vi "simulation_freq_MRC.vi"() -> ()   [LabVIEW 2014] (continued)
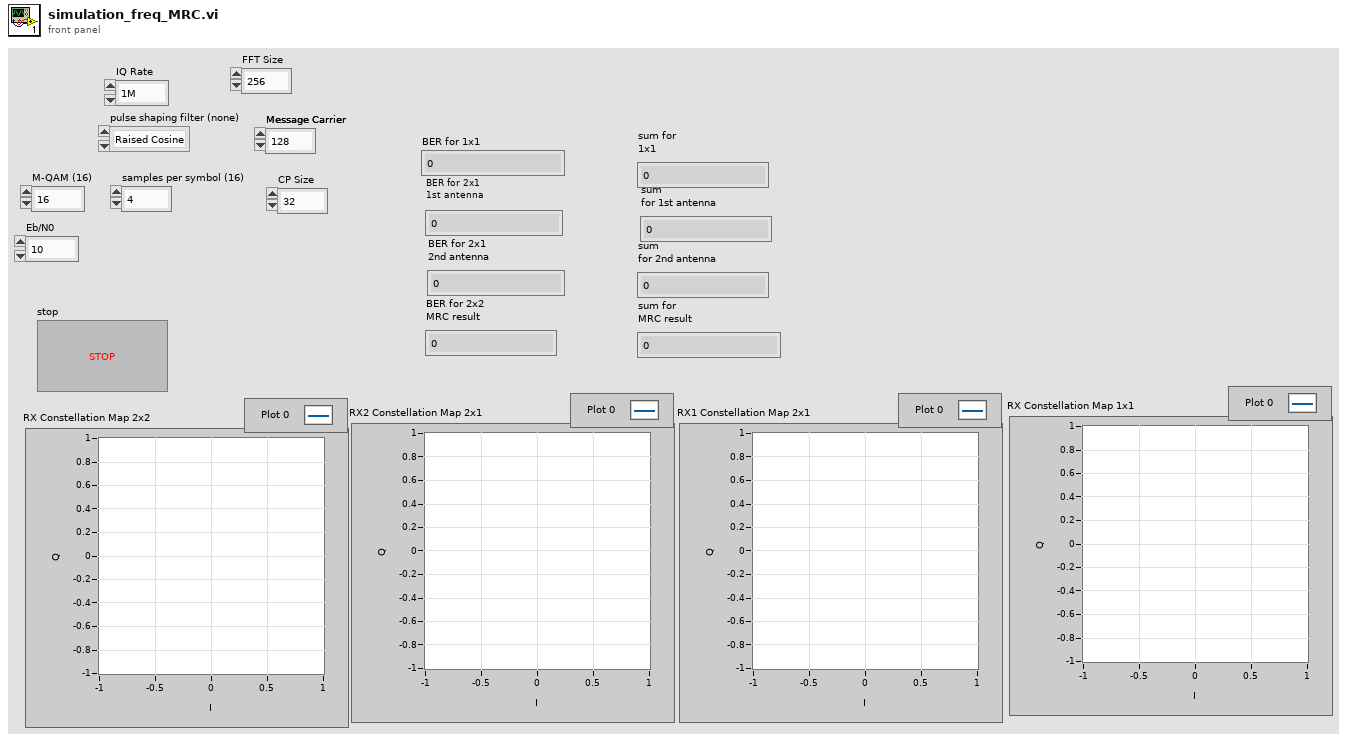
[diagram p1: front panel]
types:
  T1 = enum16{"none", "Raised Cosine", "Root Raised Cos", "Gaussian"}
  T2 = enum16{"FSK", "PSK", "QAM", "MSK", "PAM", "ASK", "CPM"}
  T3 = cluster{"samples per symbol (16)":i32, "symbol map":cdb[]}
  T4 = typedef "niAMT.lvlib/Complex Data Waveform.ctl" = cluster{"t0":dbl, "dt":dbl, "Y":cdb[]}
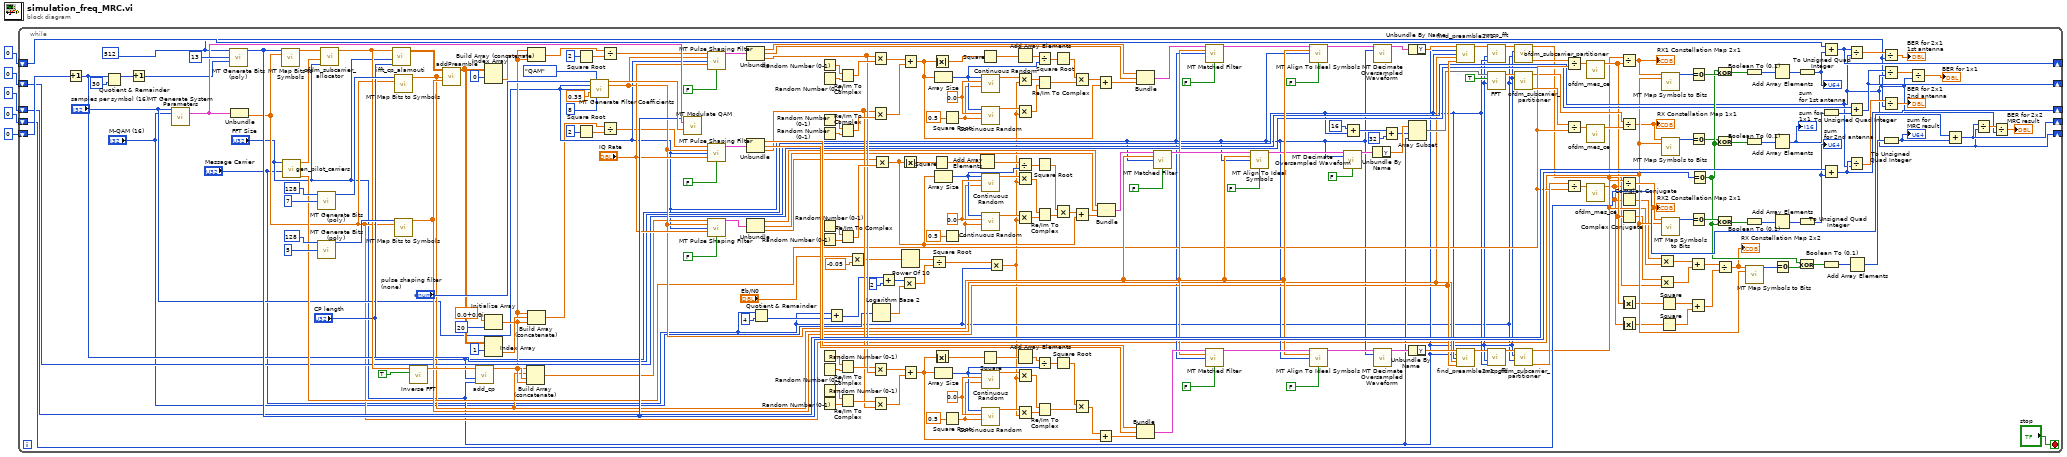
[diagram p0: block diagram]
diagram:
  n1 = while {
    shift-right: [w130] -> _
    shift-left: u64 0 -> [w214]
    shift-right: [w70] -> _
    shift-left: u64 0 -> [w215]
    shift-right: [w133] -> _
    shift-left: u64 0 -> [w178]
    shift-right: [w127] -> _
    shift-left: u64 0 -> [w177]
    shift-right: [w71] -> _
    shift-left: u64 0 -> [w72]
    stop <- "stop" stop-if-true
    w6 = 512
    w109 = 0.0 ("mean")
    w157 = 0.0 ("mean")
    w174 = 0.0 ("mean")
    n2 = Increment(x=w215) -> (x+1=w70:u64)
    n3 = Quotient & Remainder(x=w70, y=30) -> (x-y*floor(x/y)=w124:u64)  [unwired: 1 out]
    n4 = Increment(x=w124) -> (x+1=w123:u64)
    n5 = call-poly <vilib>:"MT Generate System Parameters.vi"("samples per symbol (16)"="samples per symbol (16)", "M-QAM (16)"="M-QAM (16)") -> ("QAM system parameters"=w253:T3)  [unwired: 11 in, 2 out]
    n6 = call-poly <vilib>:"MT Generate Bits (poly).vi"("total bits (128)"=w6, "PN sequence order (9)"=13, "seed in (0xD6BF7DF2)"=w123) -> ("output bit stream"=w239:i8[])  [unwired: 10 in, 2 out]
    n7 = Unbundle(w253) -> ("symbol map"=w51:cdb[])  [unwired: 1 out]
    n8 = call-poly <vilib>:"MT Map Bits to Symbols.vi"("input bit stream"=w239, "symbol map"=w51) -> ("symbols"=w250:cdb[])  [unwired: 12 in, 1 out]
    n9 = call "gen_pilot_carriers.vi"("message carrier"="Message Carrier", "FFT size"="FFT Size") -> ("RX pilot carriers"=w83:cdb[], "TX pilot carriers"=w249:cdb[])  [unwired: 8 in]
    n10 = call-poly <vilib>:"MT Generate Bits (poly).vi"("total bits (128)"=128, "PN sequence order (9)"=7) -> ("output bit stream"=w248:i8[])  [unwired: 11 in, 2 out]
    n11 = call-poly <vilib>:"MT Generate Bits (poly).vi"("total bits (128)"=128, "PN sequence order (9)"=5) -> ("output bit stream"=w247:i8[])  [unwired: 11 in, 2 out]
    n12 = call "ofdm_subcarrier_allocator.vi"("fft size"="FFT Size", "pilot symbol"=w249, "message symbol"=w250) -> ("OFDM symbol"=w122:cdb[])  [unwired: 8 in]
    n13 = call "ifft_cp_alamouti.vi"("CP Length"="CP length", "FFT Size"="FFT Size", "Modulated Stream"=w122) -> ("Baseband Streams"=w255:cdb[][])  [unwired: 8 in]
    n14 = call-poly <vilib>:"MT Map Bits to Symbols.vi"("input bit stream"=w248, "symbol map"=w51) -> ("symbols"=w58:cdb[])  [unwired: 12 in, 1 out]
    n15 = call-poly <vilib>:"MT Map Bits to Symbols.vi"("input bit stream"=w247, "symbol map"=w51) -> ("symbols"=w85:cdb[])  [unwired: 12 in, 1 out]
    n16 = call-poly <vilib>:"Inverse FFT.vi"("shift?"=TRUE, "FFT {X}"=w122) -> ("X"=w120:cdb[])  [unwired: 8 in, 1 out]
    n17 = call "addPreamble.vi"("Input Symbol Stream"=w255, "Training Sequence"=w58, "Training Sequence 2"=w85) -> ("Output Transmit \nPackets"=w243:cdb[][])  [unwired: 11 in, 1 out]
    n18 = call "add_cp.vi"("FFT size"="FFT Size", "CP length"="CP length", "time_samples"=w120) -> ("cp ofdm symbol"=w119:cdb[])  [unwired: 8 in]
    n19 = Initialize Array(cdb 0.0+0.0i ("element"), 20 ("dimension size")) -> (w59:cdb[])
    n20 = Index Array(array=w243, index (row)=0) -> (element=w218:cdb[])  [unwired: 1 in]
    n21 = Index Array(array=w243, index (row)=1) -> (element=w217:cdb[])  [unwired: 1 in]
    n22 = Build Array (concatenate)(w59, w58, w119, w59) -> (w65:cdb[])
    n23 = Build Array (concatenate)(w59, w218, w59) -> (w32:cdb[])
    n24 = Build Array (concatenate)(w59, w217, w59) -> (w30:cdb[])
    n25 = Square Root(x=2) -> (sqrt(x)=w28:dbl)
    n26 = Square Root(x=2) -> (sqrt(x)=w27:dbl)
    n27 = call <vilib>:"MT Generate Filter Coefficients.vi"("pulse shaping filter (none)"="pulse shaping filter (none)", "modulation type"=T2."QAM", "pulse shaping samples per symbol (16)"="samples per symbol (16)", "matched samples per symbol (16)"="samples per symbol (16)", "filter parameter"=0.35, "filter length (symbols)"=8) -> ("pulse shaping filter coefficients"=w251:dbl[], "matched filter coefficients"=w88:dbl[])  [unwired: 7 in, 1 out]
    n28 = Divide(x=w32, y=w28) -> (x/y=w31:cdb[])
    n29 = Divide(x=w30, y=w27) -> (x/y=w29:cdb[])
    n30 = call <vilib>:"MT Modulate QAM.vi"("input bit stream"=w239, "QAM system parameters"=w253, "pulse shaping filter coefficients"=w251) -> ()  [unwired: 10 in, 3 out]
    n31 = call-poly <vilib>:"MT Pulse Shaping Filter.vi"("symbols"=w31, "pulse shaping filter coefficients"=w88, "samples per symbol (16)"="samples per symbol (16)", "symbol rate (Hz)"="IQ Rate", "reset? (T)"=FALSE) -> ("output complex waveform"=w203:T4)  [unwired: 9 in, 1 out]
    n32 = call-poly <vilib>:"MT Pulse Shaping Filter.vi"("symbols"=w29, "pulse shaping filter coefficients"=w88, "samples per symbol (16)"="samples per symbol (16)", "symbol rate (Hz)"="IQ Rate", "reset? (T)"=FALSE) -> ("output complex waveform"=w202:T4)  [unwired: 9 in, 1 out]
    n33 = call-poly <vilib>:"MT Pulse Shaping Filter.vi"("symbols"=w65, "pulse shaping filter coefficients"=w88, "samples per symbol (16)"="samples per symbol (16)", "symbol rate (Hz)"="IQ Rate", "reset? (T)"=FALSE) -> ("output complex waveform"=w67:T4)  [unwired: 9 in, 1 out]
    n34 = Unbundle(w203) -> ("t0"=w204:dbl, "dt"=w205:dbl, "Y"=w115:cdb[])
    n35 = Unbundle(w202) -> ("t0"=w206:dbl, "dt"=w207:dbl, "Y"=w112:cdb[])
    n36 = Unbundle(w67) -> ("t0"=w93:dbl, "dt"=w92:dbl, "Y"=w110:cdb[])
    n37 = Quotient & Remainder(x="Message Carrier", y=4) -> (floor(x/y)=w19:u32)  [unwired: 1 out]
    n38 = Random Number (0-1)() -> (number: 0 to 1=w193:dbl)
    n39 = Random Number (0-1)() -> (number: 0 to 1=w192:dbl)
    n40 = Random Number (0-1)() -> (number: 0 to 1=w190:dbl)
    n41 = Random Number (0-1)() -> (number: 0 to 1=w189:dbl)
    n42 = Random Number (0-1)() -> (number: 0 to 1=w117:dbl)
    n43 = Random Number (0-1)() -> (number: 0 to 1=w111:dbl)
    n44 = Random Number (0-1)() -> (number: 0 to 1=w195:dbl)
    n45 = Random Number (0-1)() -> (number: 0 to 1=w194:dbl)
    n46 = Random Number (0-1)() -> (number: 0 to 1=w197:dbl)
    n47 = Random Number (0-1)() -> (number: 0 to 1=w196:dbl)
    n48 = Add(x="Message Carrier", y=w19) -> (x+y=w18:u32)
    n49 = Re/Im To Complex(1:w192, 2:w193) -> (0:w191:cdb)
    n50 = Re/Im To Complex(1:w189, 2:w190) -> (0:w188:cdb)
    n51 = Re/Im To Complex(1:w111, 2:w117) -> (0:w116:cdb)
    n52 = Re/Im To Complex(1:w194, 2:w195) -> (0:w114:cdb)
    n53 = Re/Im To Complex(1:w196, 2:w197) -> (0:w113:cdb)
    n54 = Multiply(x="Eb/N0", y=-0.05) -> (x*y=w8:dbl)
    n55 = Multiply(x=w115, y=w191) -> (x*y=w208:cdb[])
    n56 = Multiply(x=w112, y=w188) -> (x*y=w209:cdb[])
    n57 = Multiply(x=w114, y=w115) -> (x*y=w210:cdb[])
    n58 = Multiply(x=w113, y=w112) -> (x*y=w211:cdb[])
    n59 = Logarithm Base 2(1:"M-QAM (16)") -> (0:w15:dbl)
    n60 = Multiply(x=w110, y=w116) -> (x*y=w94:cdb[])
    n61 = Add(x=w18, y=2) -> (x+y=w16:u32)
    n62 = Multiply(x=w16, y=w15) -> (x*y=w13:dbl)
    n63 = Absolute Value(x=w94) -> (abs(x)=w104:dbl[])
    n64 = Add(x=w208, y=w209) -> (x+y=w142:cdb[])
    n65 = Power Of 10(x=w8) -> (10^x=w21:dbl)
    n66 = Add(x=w210, y=w211) -> (x+y=w159:cdb[])
    n67 = Divide(x=w21, y=w13) -> (x/y=w12:dbl)
    n68 = Square(x=w104) -> (x^2=w103:dbl[])
    n69 = Absolute Value(x=w142) -> (abs(x)=w152:dbl[])
    n70 = Absolute Value(x=w159) -> (abs(x)=w169:dbl[])
    n71 = Array Size(array=w142) -> (size(s)=w149:i32)
    n72 = Array Size(array=w94) -> (size(s)=w101:i32)
    n73 = Array Size(array=w159) -> (size(s)=w166:i32)
    n74 = Square Root(x=0.5 ("std")) -> (sqrt(x)=w143:dbl)
    n75 = Square Root(x=0.5 ("std")) -> (sqrt(x)=w95:dbl)
    n76 = Square Root(x=0.5 ("std")) -> (sqrt(x)=w160:dbl)
    n77 = Add Array Elements(numeric array=w103) -> (sum=w102:dbl)
    n78 = Square(x=w152) -> (x^2=w151:dbl[])
    n79 = Square(x=w169) -> (x^2=w168:dbl[])
    n80 = call-poly <vilib>:"Continuous Random.vi"("std"=w143, "mean"=w157, "samples"=w149) -> ("normal random data"=w155:dbl[])  [unwired: 7 in, 1 out]
    n81 = call-poly <vilib>:"Continuous Random.vi"("std"=w143, "mean"=w157, "samples"=w149) -> ("normal random data"=w156:dbl[])  [unwired: 7 in, 1 out]
    n82 = call-poly <vilib>:"Continuous Random.vi"("std"=w95, "mean"=w109, "samples"=w101) -> ("normal random data"=w107:dbl[])  [unwired: 7 in, 1 out]
    n83 = call-poly <vilib>:"Continuous Random.vi"("std"=w95, "mean"=w109, "samples"=w101) -> ("normal random data"=w108:dbl[])  [unwired: 7 in, 1 out]
    n84 = call-poly <vilib>:"Continuous Random.vi"("std"=w160, "mean"=w174, "samples"=w166) -> ("normal random data"=w172:dbl[])  [unwired: 7 in, 1 out]
    n85 = call-poly <vilib>:"Continuous Random.vi"("std"=w160, "mean"=w174, "samples"=w166) -> ("normal random data"=w173:dbl[])  [unwired: 7 in, 1 out]
    n86 = Multiply(x=w12, y="Message Carrier") -> (x*y=w10:dbl)
    n87 = Add Array Elements(numeric array=w151) -> (sum=w150:dbl)
    n88 = Multiply(x=w155, y=w10) -> (x*y=w154:dbl[])
    n89 = Multiply(x=w156, y=w10) -> (x*y=w153:dbl[])
    n90 = Divide(x=w102, y=w101) -> (x/y=w100:dbl)
    n91 = Multiply(x=w107, y=w10) -> (x*y=w106:dbl[])
    n92 = Multiply(x=w108, y=w10) -> (x*y=w105:dbl[])
    n93 = Add Array Elements(numeric array=w168) -> (sum=w167:dbl)
    n94 = Multiply(x=w172, y=w10) -> (x*y=w171:dbl[])
    n95 = Multiply(x=w173, y=w10) -> (x*y=w170:dbl[])
    n96 = Divide(x=w150, y=w149) -> (x/y=w148:dbl)
    n97 = Re/Im To Complex(1:w153, 2:w154) -> (0:w146:cdb[])
    n98 = Square Root(x=w100) -> (sqrt(x)=w99:dbl)
    n99 = Re/Im To Complex(1:w105, 2:w106) -> (0:w98:cdb[])
    n100 = Divide(x=w167, y=w166) -> (x/y=w165:dbl)
    n101 = Re/Im To Complex(1:w170, 2:w171) -> (0:w163:cdb[])
    n102 = Square Root(x=w148) -> (sqrt(x)=w147:dbl)
    n103 = Multiply(x=w99, y=w98) -> (x*y=w97:cdb[])
    n104 = Square Root(x=w165) -> (sqrt(x)=w164:dbl)
    n105 = Multiply(x=w147, y=w146) -> (x*y=w145:cdb[])
    n106 = Add(x=w97, y=w94) -> (x+y=w91:cdb[])
    n107 = Multiply(x=w164, y=w163) -> (x*y=w162:cdb[])
    n108 = Add(x=w145, y=w142) -> (x+y=w141:cdb[])
    n109 = Add(x=w162, y=w159) -> (x+y=w158:cdb[])
    n110 = Bundle("t0"=w93, "dt"=w92, w91) -> (w66:cluster{"t0":dbl, "dt":dbl, cdb[]})  [unwired: 1 in]
    n111 = Bundle("t0"=w204, "dt"=w205, w141) -> (w175:cluster{"t0":dbl, "dt":dbl, cdb[]})  [unwired: 1 in]
    n112 = Bundle("t0"=w206, "dt"=w207, w158) -> (w176:cluster{"t0":dbl, "dt":dbl, cdb[]})  [unwired: 1 in]
    n113 = call-poly <vilib>:"MT Matched Filter.vi"("input complex waveform"=w66, "matched filter coefficients"=w88, "samples per symbol (16)"="samples per symbol (16)", "reset? (T)"=FALSE) -> ("output complex waveform"=w89:T4)  [unwired: 10 in, 1 out]
    n114 = call-poly <vilib>:"MT Matched Filter.vi"("input complex waveform"=w175, "matched filter coefficients"=w88, "samples per symbol (16)"="samples per symbol (16)", "reset? (T)"=FALSE) -> ("output complex waveform"=w235:T4)  [unwired: 10 in, 1 out]
    n115 = call-poly <vilib>:"MT Matched Filter.vi"("input complex waveform"=w176, "matched filter coefficients"=w88, "samples per symbol (16)"="samples per symbol (16)", "reset? (T)"=FALSE) -> ("output complex waveform"=w233:T4)  [unwired: 10 in, 1 out]
    n116 = call-poly <vilib>:"MT Align To Ideal Symbols.vi"("input complex waveform"=w89, "matched filter coefficients"=w88, "samples per symbol (16)"="samples per symbol (16)", "reset? (T)"=FALSE) -> ("output complex waveform"=w87:T4)  [unwired: 9 in, 2 out]
    n117 = call-poly <vilib>:"MT Align To Ideal Symbols.vi"("input complex waveform"=w235, "matched filter coefficients"=w88, "samples per symbol (16)"="samples per symbol (16)", "reset? (T)"=FALSE) -> ("output complex waveform"=w234:T4)  [unwired: 9 in, 2 out]
    n118 = call-poly <vilib>:"MT Align To Ideal Symbols.vi"("input complex waveform"=w233, "matched filter coefficients"=w88, "samples per symbol (16)"="samples per symbol (16)", "reset? (T)"=FALSE) -> ("output complex waveform"=w232:T4)  [unwired: 9 in, 2 out]
    n119 = call <vilib>:"MT Decimate Oversampled Waveform.vi"("input complex waveform"=w87, "decimation factor"="samples per symbol (16)", "reset? (T)"=FALSE) -> ("output complex waveform"=w86:T4)  [unwired: 11 in, 1 out]
    n120 = Add(x=u32 16, y="CP length") -> (x+y=w56:u32)
    n121 = Unbundle By Name(w86) -> ("Y"=w64:cdb[])
    n122 = call <vilib>:"MT Decimate Oversampled Waveform.vi"("input complex waveform"=w234, "decimation factor"="samples per symbol (16)") -> ("output complex waveform"=w231:T4)  [unwired: 12 in, 1 out]
    n123 = call <vilib>:"MT Decimate Oversampled Waveform.vi"("input complex waveform"=w232, "decimation factor"="samples per symbol (16)") -> ("output complex waveform"=w230:T4)  [unwired: 12 in, 1 out]
    n124 = Add(x=w56, y=32) -> (x+y=w57:u32)
    n125 = Unbundle By Name(w231) -> ("Y"=w212:cdb[])
    n126 = Array Subset(array=w64, index=w57, length="FFT Size") -> (w62:cdb[])
    n127 = Unbundle By Name(w230) -> ("Y"=w201:cdb[])
    n128 = call "find_preamble2x1.vi"("received \ntime symbol"=w212, "FFT Size"="FFT Size", "CP Length"="CP length", "1st preamble"=w58, "2nd preamble"=w85) -> ("OFDM Symbol"=w241:cdb[])  [unwired: 10 in]
    n129 = call "find_preamble2x1.vi"("received \ntime symbol"=w201, "FFT Size"="FFT Size", "CP Length"="CP length", "1st preamble"=w58, "2nd preamble"=w85) -> ("OFDM Symbol"=w200:cdb[])  [unwired: 10 in]
    n130 = call "rmcp_fft.vi"("CP length"="CP length", "fft size"="FFT Size", "time symbol"=w241) -> ("freq output"=w221:cdb[])  [unwired: 8 in]
    n131 = call-poly <vilib>:"FFT.vi"("FFT size"="FFT Size", "shift?"=TRUE, "X"=w62) -> ("FFT {X}"=w60:cdb[])  [unwired: 7 in, 1 out]
    n132 = call "rmcp_fft.vi"("CP length"="CP length", "fft size"="FFT Size", "time symbol"=w200) -> ("freq output"=w199:cdb[])  [unwired: 8 in]
    n133 = call "ofdm_subcarrier_partitioner.vi"("message carrier"="Message Carrier", "FFT size"="FFT Size", "received symbol"=w221) -> ("pilot subcarriers"=w244:cdb[], "message subcarriers"=w39:cdb[])  [unwired: 7 in]
    n134 = call "ofdm_subcarrier_partitioner.vi"("message carrier"="Message Carrier", "FFT size"="FFT Size", "received symbol"=w60) -> ("pilot subcarriers"=w84:cdb[], "message subcarriers"=w80:cdb[])  [unwired: 7 in]
    n135 = call "ofdm_subcarrier_partitioner.vi"("message carrier"="Message Carrier", "FFT size"="FFT Size", "received symbol"=w199) -> ("pilot subcarriers"=w198:cdb[], "message subcarriers"=w40:cdb[])  [unwired: 7 in]
    n136 = Divide(x=w244, y=w83) -> (x/y=w187:cdb[])
    n137 = Divide(x=w84, y=w83) -> (x/y=w82:cdb[])
    n138 = Divide(x=w198, y=w83) -> (x/y=w134:cdb[])
    n139 = call "ofdm_mes_ce.vi"("ZF \nchannel \nestimates"=w187) -> ("interpolated\n mes carrier CE"=w43:cdb[])  [unwired: 10 in]
    n140 = call "ofdm_mes_ce.vi"("ZF \nchannel \nestimates"=w82) -> ("interpolated\n mes carrier CE"=w81:cdb[])  [unwired: 10 in]
    n141 = call "ofdm_mes_ce.vi"("ZF \nchannel \nestimates"=w134) -> ("interpolated\n mes carrier CE"=w34:cdb[])  [unwired: 10 in]
    n142 = Divide(x=w39, y=w43) -> (x/y=w48:cdb[])
    "RX1 Constellation Map 2x1" <- w48
    n143 = Divide(x=w80, y=w81) -> (x/y=w49:cdb[])
    "RX Constellation Map 1x1" <- w49
    n144 = Divide(x=w40, y=w34) -> (x/y=w52:cdb[])
    "RX2 Constellation Map 2x1" <- w52
    n145 = Complex Conjugate(1:w34) -> (0:w42:cdb[])
    n146 = Complex Conjugate(1:w43) -> (0:w41:cdb[])
    n147 = Absolute Value(x=w43) -> (abs(x)=w47:dbl[])
    n148 = Absolute Value(x=w34) -> (abs(x)=w46:dbl[])
    n149 = Multiply(x=w42, y=w40) -> (x*y=w38:cdb[])
    n150 = Multiply(x=w41, y=w39) -> (x*y=w37:cdb[])
    n151 = Square(x=w47) -> (x^2=w45:dbl[])
    n152 = Square(x=w46) -> (x^2=w44:dbl[])
    n153 = call-poly <vilib>:"MT Map Symbols to Bits.vi"("symbols"=w48, "symbol map"=w51) -> ("output bit stream"=w240:i8[])  [unwired: 12 in, 1 out]
    n154 = call-poly <vilib>:"MT Map Symbols to Bits.vi"("symbols"=w49, "symbol map"=w51) -> ("output bit stream"=w79:i8[])  [unwired: 12 in, 1 out]
    n155 = call-poly <vilib>:"MT Map Symbols to Bits.vi"("symbols"=w52, "symbol map"=w51) -> ("output bit stream"=w186:i8[])  [unwired: 12 in, 1 out]
    n156 = Add(x=w38, y=w37) -> (x+y=w36:cdb[])
    n157 = Add(x=w45, y=w44) -> (x+y=w33:dbl[])
    n158 = Equal To 0?(x=w240) -> (x = 0?=w238:bool[])
    n159 = Equal To 0?(x=w79) -> (x = 0?=w77:bool[])
    n160 = Equal To 0?(x=w186) -> (x = 0?=w185:bool[])
    n161 = Equal To 0?(x=w239) -> (x = 0?=w78:bool[])
    n162 = Exclusive Or(1:w238, 2:w78) -> (0:w237:bool[])
    n163 = Exclusive Or(1:w78, 2:w77) -> (0:w76:bool[])
    n164 = Exclusive Or(1:w78, 2:w185) -> (0:w181:bool[])
    n165 = Divide(x=w36, y=w33) -> (x/y=w35:cdb[])
    "RX Constellation Map 2x2" <- w35
    n166 = Boolean To (0,1)(Boolean=w237) -> (0, 1=w236:i16[])
    n167 = Boolean To (0,1)(Boolean=w76) -> (0, 1=w75:i16[])
    n168 = Boolean To (0,1)(Boolean=w181) -> (0, 1=w180:i16[])
    n169 = call-poly <vilib>:"MT Map Symbols to Bits.vi"("symbols"=w35, "symbol map"=w51) -> ("output bit stream"=w184:i8[])  [unwired: 12 in, 1 out]
    n170 = Add Array Elements(numeric array=w236) -> (sum=w139:i16)
    n171 = Add Array Elements(numeric array=w75) -> (sum=w74:i16)
    "sum for\n1x1" <- w74
    n172 = Add Array Elements(numeric array=w180) -> (sum=w137:i16)
    n173 = Equal To 0?(x=w184) -> (x = 0?=w183:bool[])
    n174 = Exclusive Or(1:w183, 2:w78) -> (0:w182:bool[])
    n175 = To Unsigned Quad Integer(1:w139) -> (0:w140:u64)
    "sum \nfor 1st antenna" <- w140
    n176 = To Unsigned Quad Integer(1:w137) -> (0:w138:u64)
    "sum \nfor 2nd antenna" <- w138
    n177 = Add(x=w214, y=w140) -> (x+y=w130:u64)
    n178 = To Unsigned Quad Integer(1:w74) -> (0:w73:u64)
    n179 = Add(x=w178, y=w138) -> (x+y=w133:u64)
    n180 = Boolean To (0,1)(Boolean=w182) -> (0, 1=w179:i16[])
    n181 = Divide(x=w130, y=w70) -> (x/y=w129:dbl)
    n182 = Add(x=w72, y=w73) -> (x+y=w71:u64)
    n183 = Divide(x=w133, y=w70) -> (x/y=w132:dbl)
    n184 = Add Array Elements(numeric array=w179) -> (sum=w136:i16)
    n185 = Divide(x=w129, y=w6) -> (x/y=→"BER for 2x1\n1st antenna":dbl)
    n186 = Divide(x=w71, y=w70) -> (x/y=w69:dbl)
    n187 = Divide(x=w132, y=w6) -> (x/y=→"BER for 2x1\n2nd antenna":dbl)
    n188 = To Unsigned Quad Integer(1:w136) -> (0:w135:u64)
    "sum for \nMRC result" <- w135
    n189 = Divide(x=w69, y=w6) -> (x/y=→"BER for 1x1":dbl)
    n190 = Add(x=w177, y=w135) -> (x+y=w127:u64)
    n191 = Divide(x=w127, y=w70) -> (x/y=w126:dbl)
    n192 = Divide(x=w126, y=w6) -> (x/y=→"BER for 2x2 \nMRC result":dbl)
  }
